vi "generateSignalByCase.vi"(5 "Reset Control":bool, 6 "detla Parametros":T2, 7 "Parametros Maximos":T2, 8 "Sound Parameters":cluster{"# samples":u32, "tiempos (ms)":dbl}, 9 "ControlCase":T1 items=["CONTROL_INITIAL_AVERAGE", "CONTROL_GENERATE_RANDOM_SIGNAL", "CONTROL_INCREMENT_MIDTIME", "CONTROL_AVERAGE_MIDTIME", "CONTROL_INITIATE_AMPLITUDE", "CONTROL_INCREMENT_AMPLITUDE", "CONTROL_AVERAGE_AMPLITUDE", "CONTROL_INITIATE_SIGMA", "CONTROL_INCREMENT_SIGMA", "CONTROL_AVERAGE_SIGMA", "CONTROL_BEST_SIGNAL", "CONTROL_ADJUST_OFF", "CONTROL_OFF"]) -> (0 "Parametros Iniciales":T2, 1 "Mejores Parametros":T2, 2 "Parametros Actuales":T2, 3 "Señal de Control OUT":dbl[](array[numeric]), 4 "Arreglo de Salida":dbl[](array[numeric]))   [LabVIEW 2010]
uses:
  CaseControl.ctl
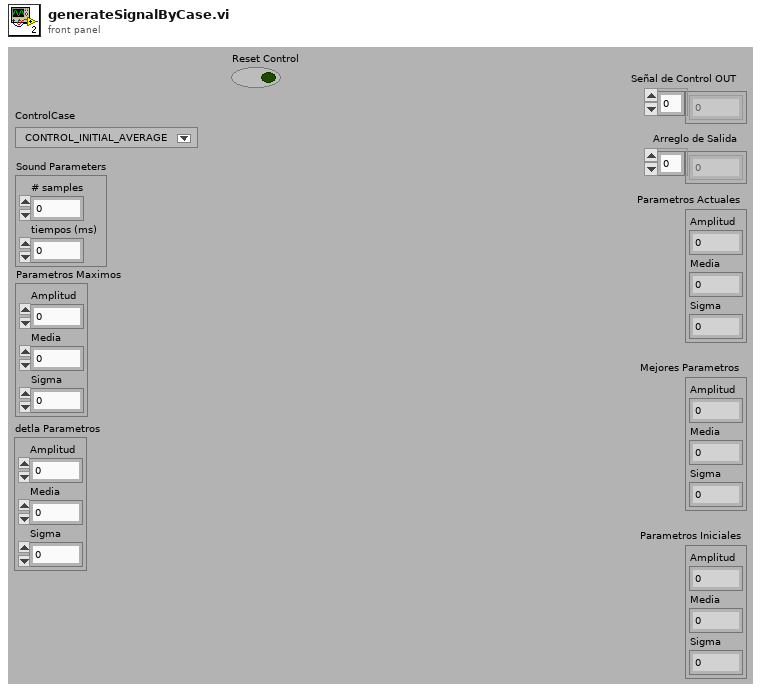
[diagram p1: front panel]
types:
  T1 = typedef "CaseControl.ctl" = u32
  T2 = cluster{"Amplitud":dbl, "Media":dbl, "Sigma":dbl}
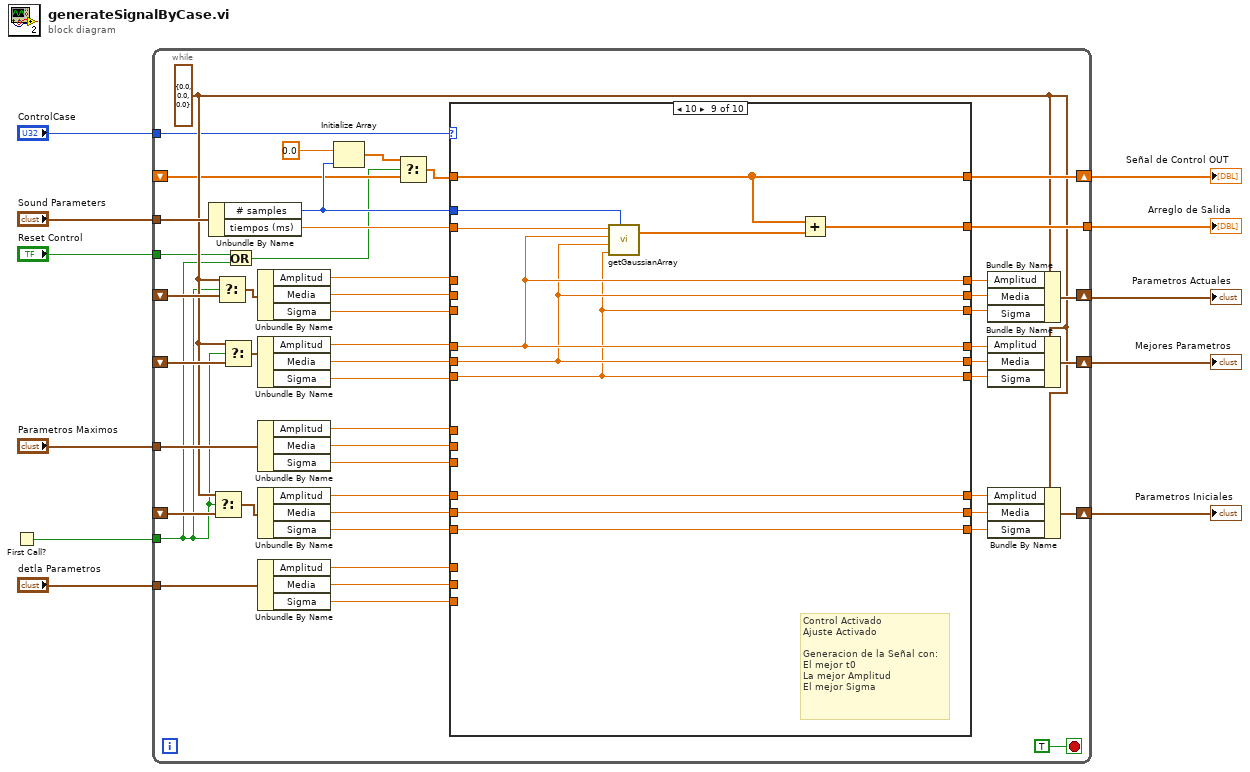
[diagram p0: block diagram]
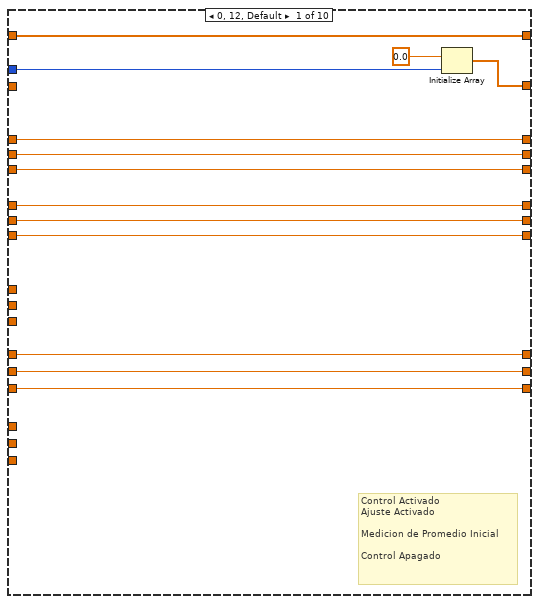
[diagram p2: hidden frame]
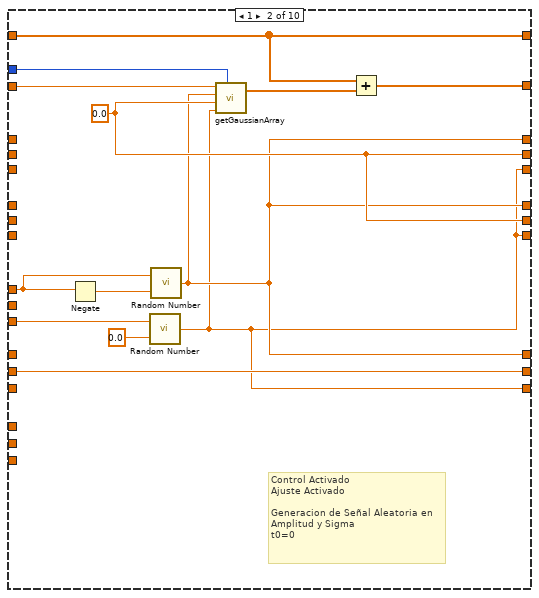
[diagram p3: hidden frame]
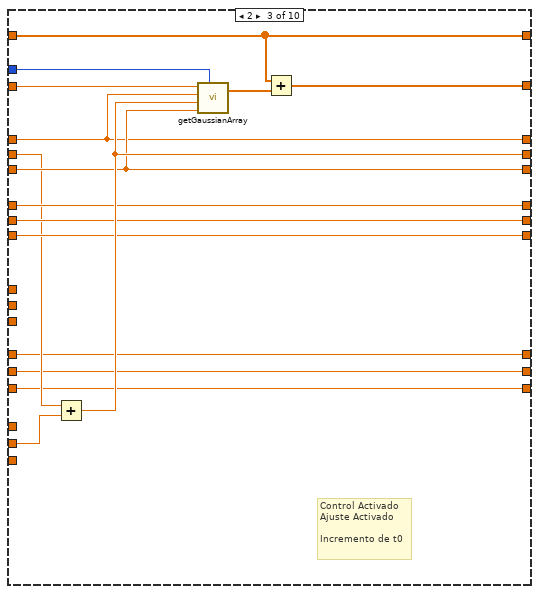
[diagram p4: hidden frame]
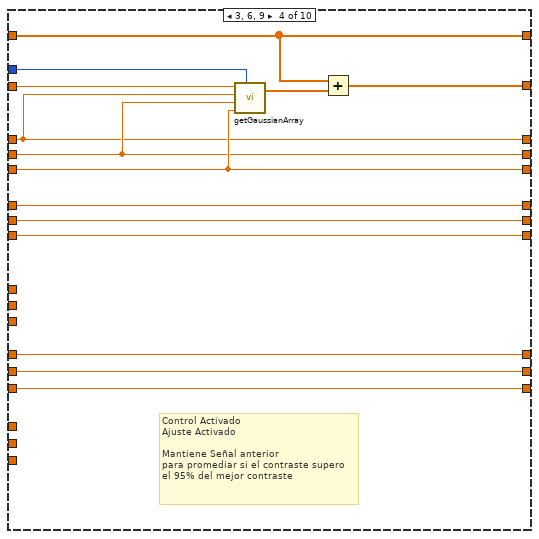
[diagram p5: hidden frame]
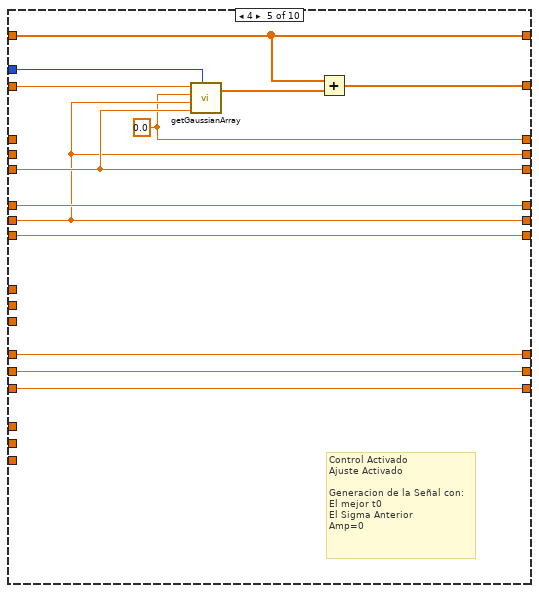
[diagram p6: hidden frame]
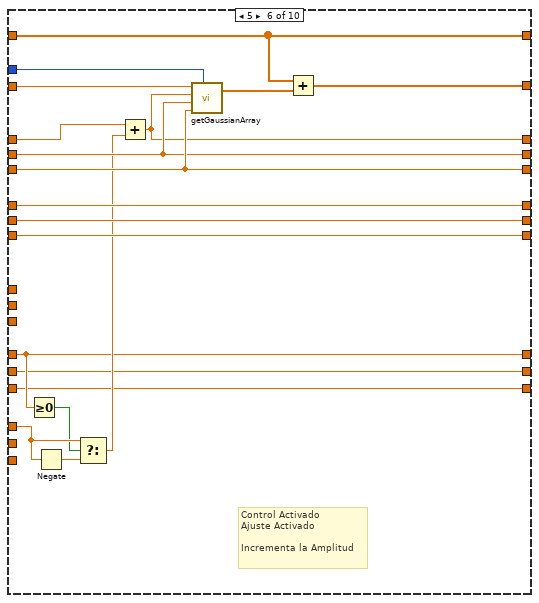
[diagram p7: hidden frame]
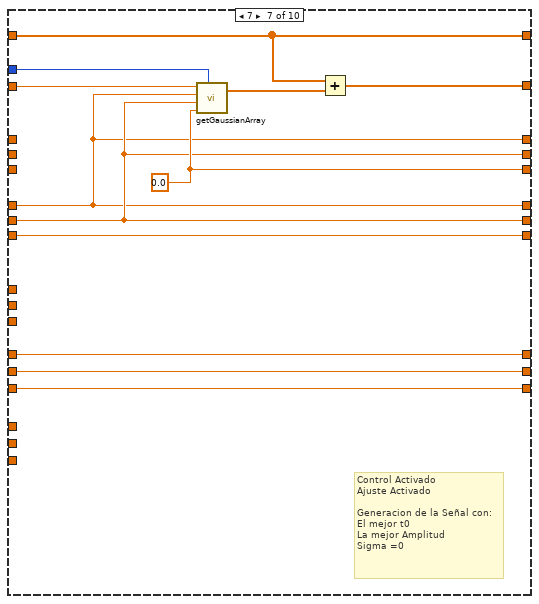
[diagram p8: hidden frame]
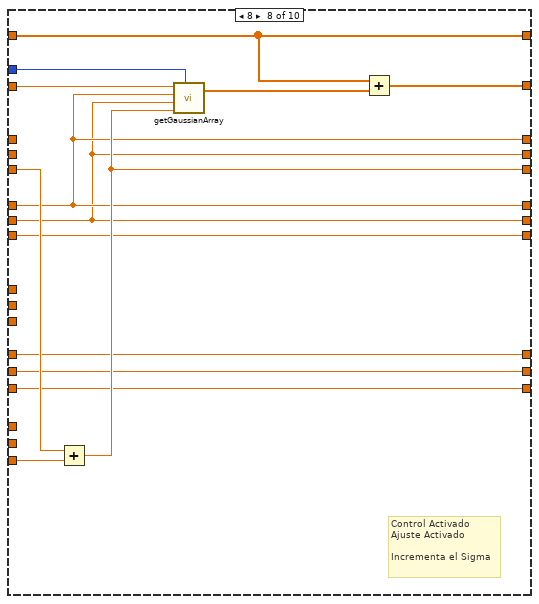
[diagram p9: hidden frame]
diagram:
  n1 = First Call?() -> (First Call?: T/F=w4:bool)
  n2 = while {
    tunnel: [w60] -> w10
    tunnel: "detla Parametros" -> [w57]
    tunnel: "Parametros Maximos" -> [w53]
    tunnel: "Sound Parameters" -> [w42]
    shift-right: [w31] -> w3
    shift-left: _ -> [w26]
    tunnel: w4 -> [w15]
    shift-right: [w40] -> w5
    shift-left: _ -> [w24]
    shift-right: [w48] -> w7
    shift-left: _ -> [w25]
    shift-right: [w61] -> w11
    shift-left: _ -> [w18]
    tunnel: "Reset Control" -> [w13]
    tunnel: "ControlCase" -> [w12]
    stop <- TRUE stop-if-true
    w23 = T2 {"Amplitud"=0.0, "Media"=0.0, "Sigma"=0.0} ("input cluster")
    n3 = Unbundle By Name(w42) -> ("# samples"=w19:u32, "tiempos (ms)"=w41:dbl)
    n4 = Select(t=w23, s=w15, f=w26) -> (s? t:f=w27:T2)
    n5 = Select(t=w23, s=w15, f=w25) -> (s? t:f=w22:T2)
    n6 = Select(t=w23, s=w15, f=w24) -> (s? t:f=w21:T2)
    n7 = Or(x=w13, y=w15) -> (x .or. y?=w14:bool)
    n8 = Unbundle By Name(w22) -> ("Amplitud"=w45:dbl, "Media"=w47:dbl, "Sigma"=w46:dbl)
    n9 = Unbundle By Name(w21) -> ("Amplitud"=w59:dbl, "Media"=w58:dbl, "Sigma"=w43:dbl)
    n10 = Unbundle By Name(w53) -> ("Amplitud"=w52:dbl, "Media"=w44:dbl, "Sigma"=w51:dbl)
    n11 = Unbundle By Name(w27) -> ("Amplitud"=w34:dbl, "Media"=w33:dbl, "Sigma"=w32:dbl)
    n12 = Unbundle By Name(w57) -> ("Amplitud"=w56:dbl, "Media"=w55:dbl, "Sigma"=w54:dbl)
    n13 = Initialize Array(0.0 ("element"), w19) -> (w17:dbl[])
    n14 = Select(t=w17, s=w14, f=w18) -> (s? t:f=w16:dbl[])
    n15 = case shown="10" w12 {
      tunnel: [w73 w83 w101 w117 w130 w149 w160 w175 w176 w196] -> w60
      tunnel: w19 -> [w74 w78 w95 w108 w123 w131 w152 w171 w182 _]
      tunnel: w41 -> [_ w79 w94 w109 w122 w132 w153 w170 w181 _]
      tunnel: w52 -> [_ w86 _ _ _ _ _ _ _ _]
      tunnel: w51 -> [_ w85 _ _ _ _ _ _ _ _]
      tunnel: [w66 w80 w103 w115 w125 w147 w151 w165 w179 w195] -> w36
      tunnel: [w68 w76 w93 w107 w121 w133 w150 w166 w180 w193] -> w50
      tunnel: [w65 w75 w102 w116 w129 w148 w161 w174 w178 w194] -> w49
      tunnel: w55 -> [_ _ w92 _ _ _ _ _ _ _]
      tunnel: w47 -> [w66 _ w91 w115 _ w147 _ _ _ w195]
      tunnel: w46 -> [w65 _ w102 w116 w129 w148 _ w169 _ w194]
      tunnel: w45 -> [w68 _ w93 w107 _ w144 _ _ _ w193]
      tunnel: w16 -> [w69 w81 w96 w110 w127 w145 w155 w173 w177 w196]
      tunnel: [w69 w81 w96 w110 w127 w145 w155 w173 w177 w196] -> w61
      tunnel: w58 -> [w63 _ w99 w113 w125 w143 w151 w165 w179 w191]
      tunnel: w59 -> [w64 _ w100 w114 w126 w141 w150 w166 w180 w192]
      tunnel: w56 -> [_ _ _ _ _ w139 _ _ _ _]
      tunnel: w54 -> [_ _ _ _ _ _ _ w168 _ _]
      tunnel: w43 -> [w62 _ w98 w112 w124 w142 w156 w167 w178 w190]
      tunnel: w44 -> [_ _ _ _ _ _ _ _ _ _]
      tunnel: [w64 w76 w100 w114 w126 w141 w150 w166 w180 w192] -> w39
      tunnel: [w63 w80 w99 w113 w125 w143 w151 w165 w179 w191] -> w38
      tunnel: [w62 w75 w98 w112 w124 w142 w156 w167 w178 w190] -> w37
      tunnel: w34 -> [w72 _ w90 w106 w120 w136 w159 w164 w186 w189]
      tunnel: w33 -> [w71 w77 w89 w105 w119 w135 w158 w163 w185 w188]
      tunnel: w32 -> [w70 _ w88 w104 w118 w134 w157 w162 w184 w187]
      tunnel: [w72 w76 w90 w106 w120 w136 w159 w164 w186 w189] -> w30
      tunnel: [w71 w77 w89 w105 w119 w135 w158 w163 w185 w188] -> w29
      tunnel: [w70 w75 w88 w104 w118 w134 w157 w162 w184 w187] -> w28
      frame 0, 12, Default {
        # "Control Activado\nAjuste Activado\n\nMedicion de Promedio Inicial\n\nControl Apagado"
        n16 = Initialize Array(0.0, w74) -> (w73:dbl[])
      }
      frame 1 {
        w80 = 0.0 ("t0 (ms)")
        # "Control Activado\nAjuste Activado\n\nGeneracion de Señal Aleatoria en\nAmplitud y Sigma\nt0=0"
        n17 = Negate(x=w86) -> (-x=w87:dbl)
        n18 = call "Random Number.vi"("Min"=0.0, "Max"=w85) -> ("Out"=w75:dbl)
        n19 = call "Random Number.vi"("Min"=w87, "Max"=w86) -> ("Out"=w76:dbl)
        n20 = call "getGaussianArray.vi"("tiempo (ms)"=w79, "Amplitud"=w76, "t0 (ms)"=w80, "Sigma (ms)"=w75, "#samples"=w78) -> ("Y out"=w82:dbl[])  [unwired: 1 out]
        n21 = Add(x=w81, y=w82) -> (x+y=w83:dbl[])
      }
      frame 2 {
        # "Control Activado\nAjuste Activado\n\nIncremento de t0"
        n22 = Add(x=w91, y=w92) -> (x+y=w103:dbl)
        n23 = call "getGaussianArray.vi"("tiempo (ms)"=w94, "Amplitud"=w93, "t0 (ms)"=w103, "Sigma (ms)"=w102, "#samples"=w95) -> ("Y out"=w97:dbl[])  [unwired: 1 out]
        n24 = Add(x=w96, y=w97) -> (x+y=w101:dbl[])
      }
      frame 3, 6, 9 {
        # "Control Activado\nAjuste Activado\n\nMantiene Señal anterior \npara promediar si el contraste supero\nel 95% del mejor contraste"
        n25 = call "getGaussianArray.vi"("tiempo (ms)"=w109, "Amplitud"=w107, "t0 (ms)"=w115, "Sigma (ms)"=w116, "#samples"=w108) -> ("Y out"=w111:dbl[])  [unwired: 1 out]
        n26 = Add(x=w110, y=w111) -> (x+y=w117:dbl[])
      }
      frame 4 {
        w121 = 0.0 ("Amplitud")
        # "Control Activado\nAjuste Activado\n\nGeneracion de la Señal con:\nEl mejor t0\nEl Sigma Anterior\nAmp=0"
        n27 = call "getGaussianArray.vi"("tiempo (ms)"=w122, "Amplitud"=w121, "t0 (ms)"=w125, "Sigma (ms)"=w129, "#samples"=w123) -> ("Y out"=w128:dbl[])  [unwired: 1 out]
        n28 = Add(x=w127, y=w128) -> (x+y=w130:dbl[])
      }
      frame 5 {
        # "Control Activado\nAjuste Activado\n\nIncrementa la Amplitud"
        n29 = Greater Or Equal To 0?(x=w136) -> (x >= 0?=w138:bool)
        n30 = Negate(x=w139) -> (-x=w140:dbl)
        n31 = Select(t=w139, s=w138, f=w140) -> (s? t:f=w137:dbl)
        n32 = Add(x=w144, y=w137) -> (x+y=w133:dbl)
        n33 = call "getGaussianArray.vi"("tiempo (ms)"=w132, "Amplitud"=w133, "t0 (ms)"=w147, "Sigma (ms)"=w148, "#samples"=w131) -> ("Y out"=w146:dbl[])  [unwired: 1 out]
        n34 = Add(x=w145, y=w146) -> (x+y=w149:dbl[])
      }
      frame 7 {
        w161 = 0.0 ("Sigma (ms)")
        # "Control Activado\nAjuste Activado\n\nGeneracion de la Señal con:\nEl mejor t0\nLa mejor Amplitud\nSigma =0"
        n35 = call "getGaussianArray.vi"("tiempo (ms)"=w153, "Amplitud"=w150, "t0 (ms)"=w151, "Sigma (ms)"=w161, "#samples"=w152) -> ("Y out"=w154:dbl[])  [unwired: 1 out]
        n36 = Add(x=w155, y=w154) -> (x+y=w160:dbl[])
      }
      frame 8 {
        # "Control Activado\nAjuste Activado\n\nIncrementa el Sigma"
        n37 = Add(x=w169, y=w168) -> (x+y=w174:dbl)
        n38 = call "getGaussianArray.vi"("tiempo (ms)"=w170, "Amplitud"=w166, "t0 (ms)"=w165, "Sigma (ms)"=w174, "#samples"=w171) -> ("Y out"=w172:dbl[])  [unwired: 1 out]
        n39 = Add(x=w173, y=w172) -> (x+y=w175:dbl[])
      }
      frame 10 {
        # "Control Activado\nAjuste Activado\n\nGeneracion de la Señal con:\nEl mejor t0\nLa mejor Amplitud\nEl mejor Sigma"
        n40 = call "getGaussianArray.vi"("tiempo (ms)"=w181, "Amplitud"=w180, "t0 (ms)"=w179, "Sigma (ms)"=w178, "#samples"=w182) -> ("Y out"=w183:dbl[])  [unwired: 1 out]
        n41 = Add(x=w177, y=w183) -> (x+y=w176:dbl[])
      }
      frame 11 {
        # "Control Activado\nAjuste desactivado"
      }
    }
    n42 = Bundle By Name(cluster=w23, "Amplitud"=w50, "Media"=w36, "Sigma"=w49) -> (w48:T2)
    n43 = Bundle By Name(cluster=w23, "Amplitud"=w39, "Media"=w38, "Sigma"=w37) -> (w40:T2)
    n44 = Bundle By Name(cluster=w23, "Amplitud"=w30, "Media"=w29, "Sigma"=w28) -> (w31:T2)
  }
  "Señal de Control OUT" <- w11
  "Arreglo de Salida" <- w10
  "Parametros Actuales" <- w7
  "Mejores Parametros" <- w5
  "Parametros Iniciales" <- w3
